vi "wait_for_pump1.vi"(8 "error in (no error)":errorcluster, 11 "HTS PORT IN":refnum<visa-resource-name>) -> (0 "error out":errorcluster, 3 "HTS PORT OUT":refnum<visa-resource-name>)   [LabVIEW 2013]
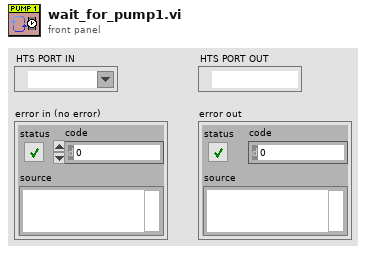
[diagram p1: front panel]
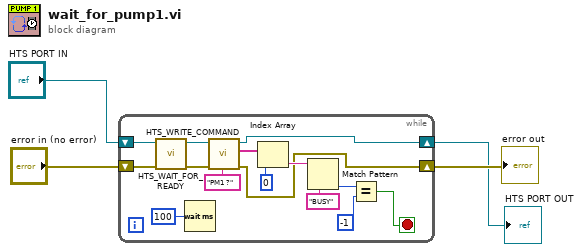
[diagram p0: block diagram]
diagram:
  n1 = while {
    shift-right: [w11] -> w1
    shift-left: "HTS PORT IN" -> [w8]
    shift-right: [w10] -> w2
    shift-left: "error in (no error)" -> [w6]
    stop <- w14 stop-if-true
    n2 = call "HTS_WAIT_FOR_READY.vi"("Error IN"=w6, "VISA resource IN"=w8) -> ("Error OUT"=w5:errorcluster, "VISA resource OUT"=w7:refnum<visa-resource-name>)  [unwired: 6 in, 2 out]
    n3 = Wait (ms)(milliseconds to wait=u32 100) -> ()  [unwired: 1 out]
    n4 = call "HTS_WRITE_COMMAND.vi"("Error IN"=w5, "Command"="PM1 ?", "HTS PORT IN"=w7) -> ("Error OUT"=w10:errorcluster, "RESPONSE"=w12:string[], "HTS PORT OUT"=w11:refnum<visa-resource-name>)  [unwired: 6 in]
    n5 = Index Array(array=w12, index=0) -> (element=w18:string)
    n6 = Match Pattern(string=w18, regular expression="BUSY") -> (offset past match=w16:i32)  [unwired: 4 out]
    n7 = Equal?(x=w16, y=-1) -> (x = y?=w14:bool)
  }
  "error out" <- w2
  "HTS PORT OUT" <- w1
